vi "LDF Exe Frame To Bus.vi"(9 "FillBitValue":u8, 10 "pFrameName":string, 11 "LDFHandle":u64) -> (2 "pFrameName out":string, 3 "function return":i32)   [LabVIEW 2010, in "ldf_parser.lvlib"]
doc: "int WINAPI LDF_ExeFrameToBus(long long LDFHandle, char* pFrameName, unsigned char FillBitValue);"
uses:
  ldf_parser.lvlib
  USB2XXX/trunk/USB2XXX/USB2XXX/vs2019/Release/USB2XXX.dll
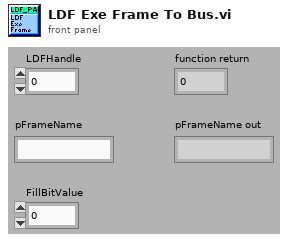
[diagram p1: front panel]
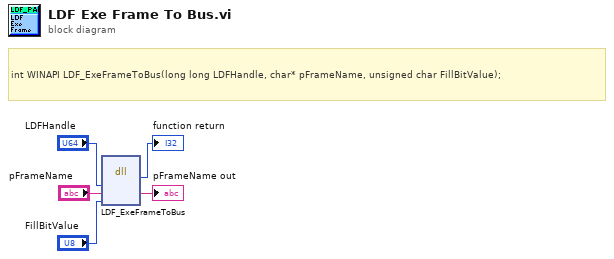
[diagram p0: block diagram]
diagram:
  # "int WINAPI LDF_ExeFrameToBus(long long LDFHandle, char* pFrameName, unsigned char FillBitValue);"
  n1 = dll-call lib="E:/Projects/USB2XXX/trunk/USB2XXX/USB2XXX/vs2019/Release/USB2XXX.*" fn="LDF_ExeFrameToBus"("LDFHandle"="LDFHandle", "pFrameName"="pFrameName", "FillBitValue"="FillBitValue") -> (→"function return":i32, "pFrameName"=→"pFrameName out":string)  [unwired: 5 in, 2 out]
